vi "Exp_ICCD_GetAuxOutProperties.vi"(8 "error in (no error)":errorcluster, 11 "LightField Automation in":refnum<class "LightField Automation.lvclass">) -> (0 "error out":errorcluster, 1 "Aux Out Width (ns)":dbl, 2 "AuxOut Delay (ns)":dbl, 3 "LightField Automation out":refnum<class "LightField Automation.lvclass">)   [LabVIEW 2018, in "LightField Automation.lvclass"]
uses:
  LightField Automation.lvclass
  C:/Users/xw9/Desktop/Turbulence program/SourceDistribution/PrincetonInstruments.LightFieldAddInSupportServices.dll
  PrincetonInstruments.LightFieldAddInSupportServices.dll
  C:/Users/xw9/Desktop/Turbulence program/SourceDistribution/PrincetonInstruments.LightFieldViewV3.dll
  PrincetonInstruments.LightFieldViewV3.dll
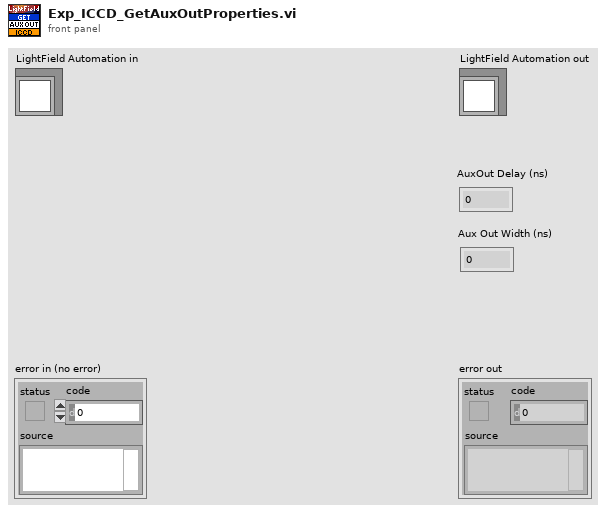
[diagram p1: front panel]
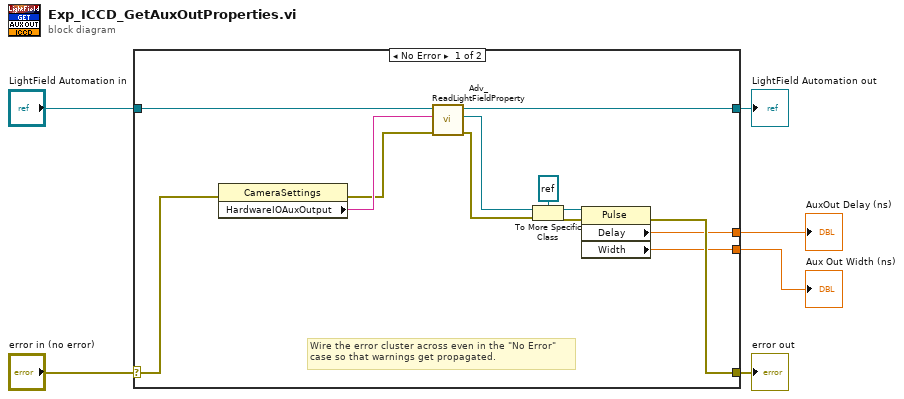
[diagram p0: block diagram]
diagram:
  n1 = case shown="No Error" "error in (no error)" {
    selector: "error in (no error)" -> [w19 w21]
    tunnel: [w15 w21] -> w5
    tunnel: [w12 w20] -> w3
    tunnel: "LightField Automation in" -> [w11 w20]
    tunnel: [w14 _] -> w2
    tunnel: [w13 _] -> w1
    frame No Error {
      # "Wire the error cluster across even in the \"No Error\"\ncase so that warnings get propagated."
      n2 = property class="CameraSettings"(error in=w19) -> (error out=w9:errorcluster, "HardwareIOAuxOutput"=w10:string)  [unwired: 1 in, 1 out]
      n3 = call "Adv_ReadLightFieldProperty.vi"("error in (no error)"=w9, "setting"=w10, "LightField Automation in"=w11) -> ("error out"=w8:errorcluster, "value"=w7:refnum<k24>, "LightField Automation out"=w12:refnum<class "LightField Automation.lvclass">)  [unwired: 6 in]
      n4 = To More Specific Class(target class=refnum<k24> refnum ("reference out"), reference=w7, error in=w8) -> (specific class reference=w17:refnum<k24>, error out=w16:errorcluster)
      n5 = property class="Pulse"(reference=w17, error in=w16) -> (error out=w15:errorcluster, "Delay"=w14:dbl, "Width"=w13:dbl)  [unwired: 1 out]
    }
    frame Error {
    }
  }
  "error out" <- w5
  "LightField Automation out" <- w3
  "AuxOut Delay (ns)" <- w2
  "Aux Out Width (ns)" <- w1
